vi "ScanPath.vi"(0 "Scan parameters":T2, 1 "Axis parameters":cluster{"X axis":dbl[], "Z axis":dbl[]}={"X axis"=[1.0, 0.0, 0.0], "Z axis"=[0.0, 0.0, 1.0]}, 2 "Position":dbl[](array[numeric]), 3 "error in (no error)":errorcluster) -> (4 "Scanmode":enum16{"X", "Y", "Z", "YZ", "XZ", "XY"}(ring), 5 "ScanPath":T1, 6 "Scan Ready":bool, 7 "Ticks":dbl[][](array[numeric]), 8 "error out":errorcluster)   [LabVIEW 2016]
uses:
  <vilib>/Analysis/Matrix/Datatypes/RealMatrix.ctl
  <vilib>/Analysis/Matrix/NI_Matrix.lvlib
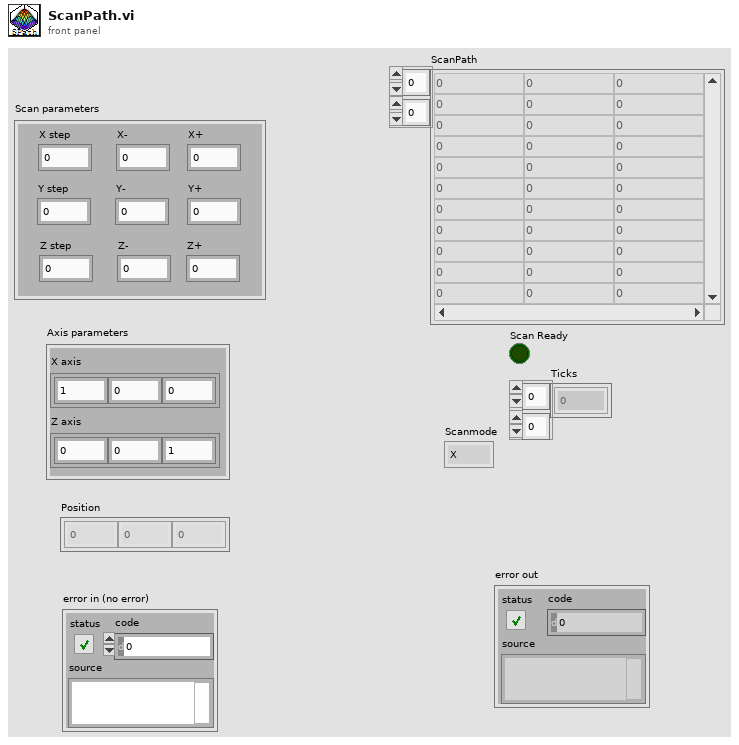
[diagram p1: front panel]
types:
  T1 = typedef "NI_Matrix.lvlib/RealMatrix.ctl" = dbl[][]
  T2 = cluster{"X-":dbl, "X step":dbl, "Y-":dbl, "Y step":dbl, "Z-":dbl, "Z step":dbl, "Z+":dbl, "X+":dbl, "Y+":dbl}
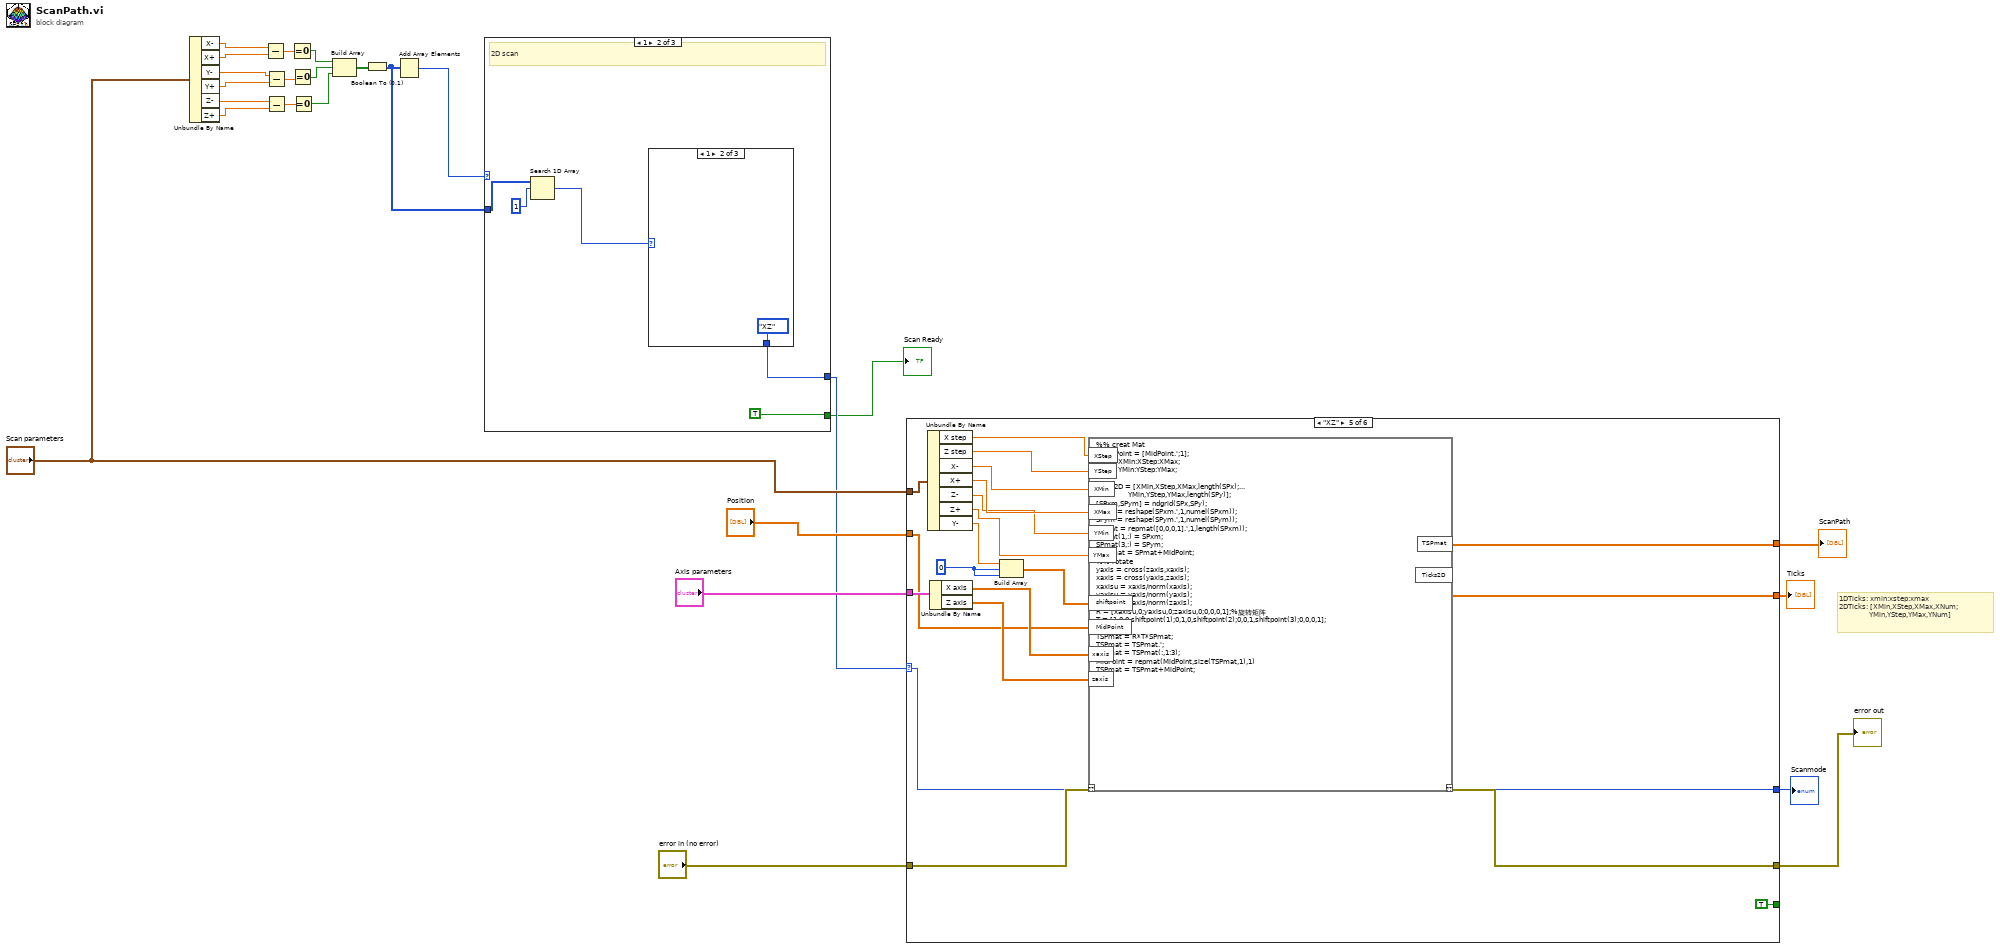
[diagram p0: block diagram]
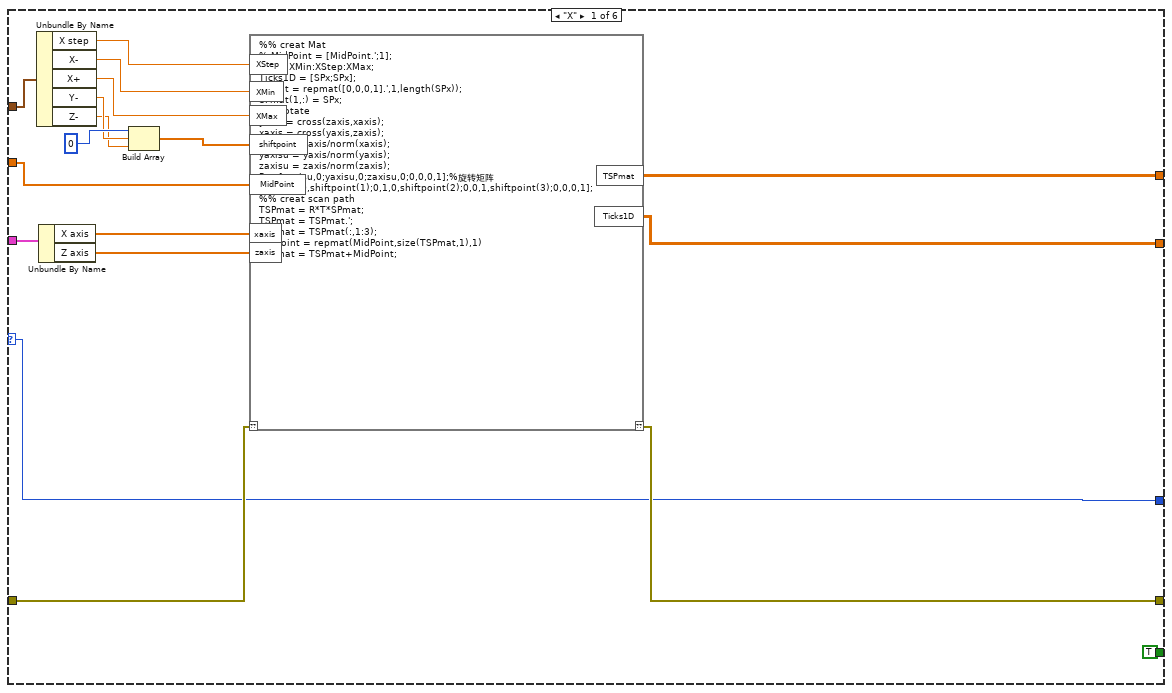
[diagram p2: hidden frame]
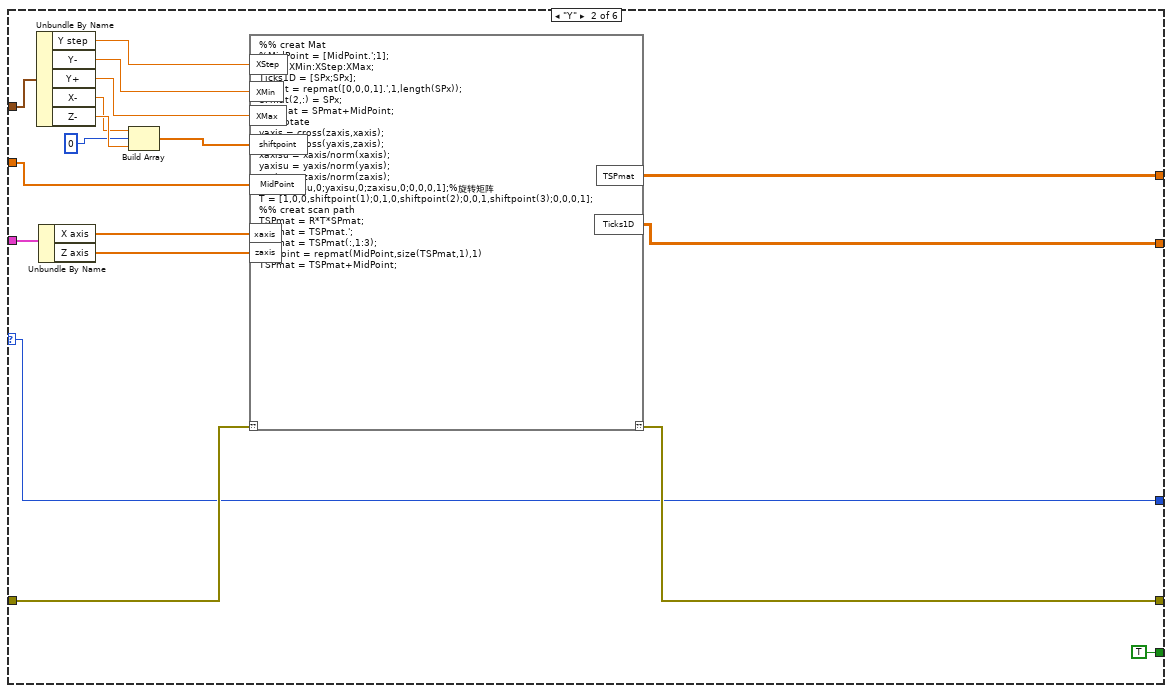
[diagram p3: hidden frame]
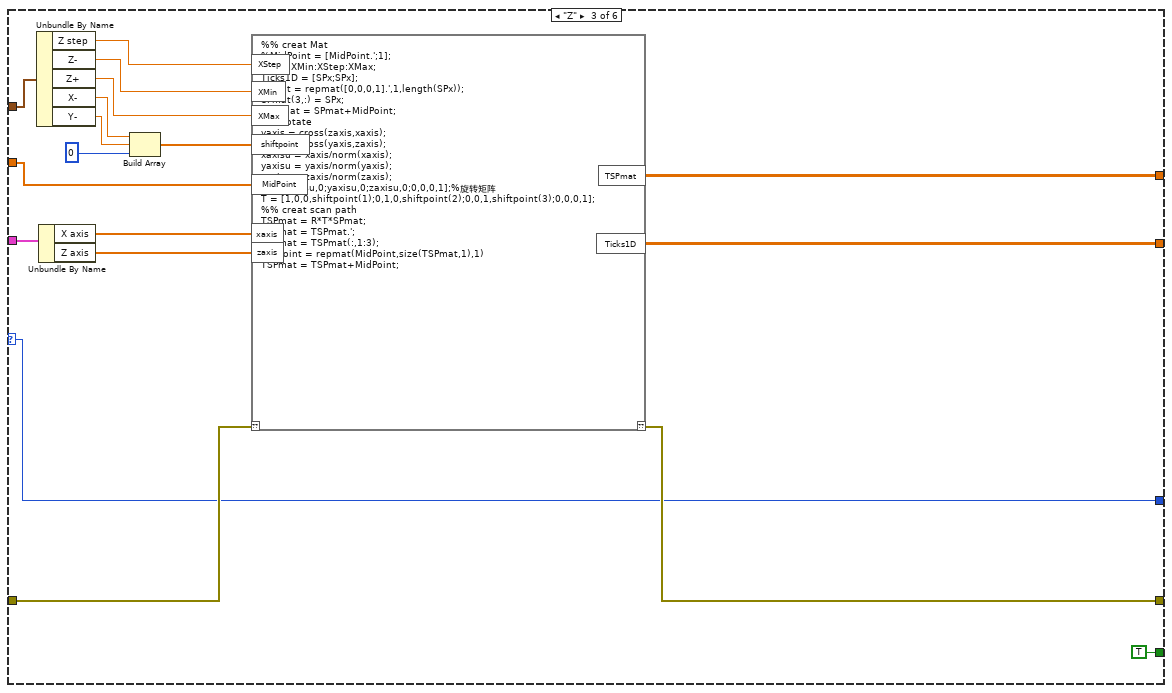
[diagram p4: hidden frame]
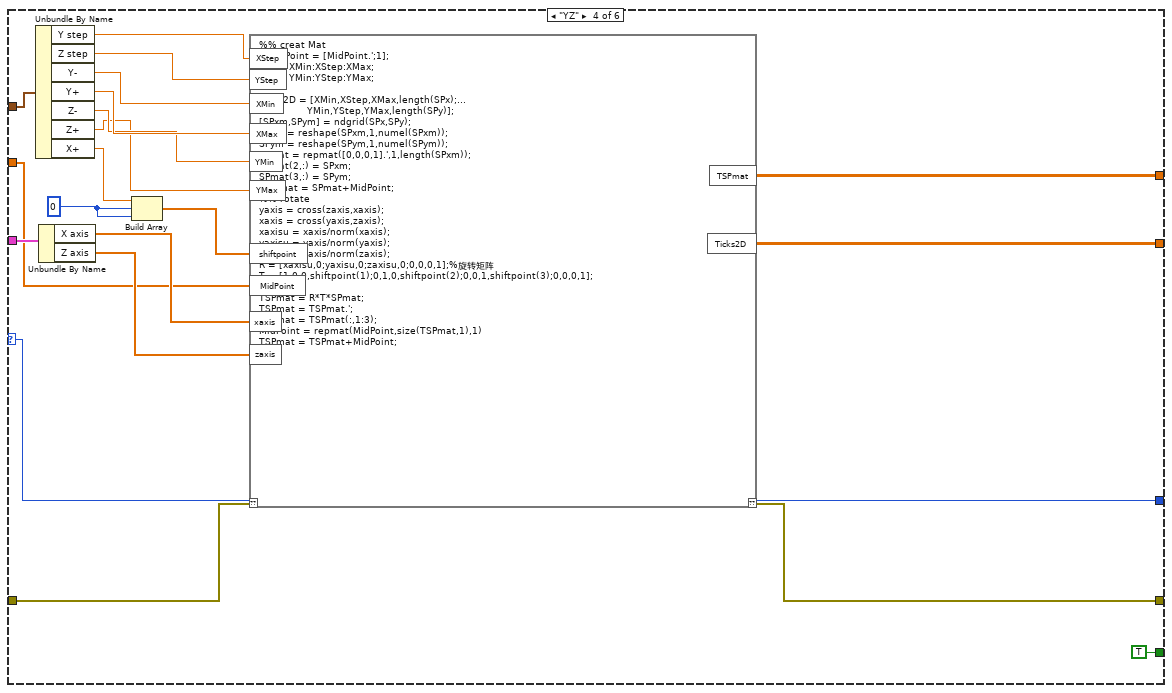
[diagram p5: hidden frame]
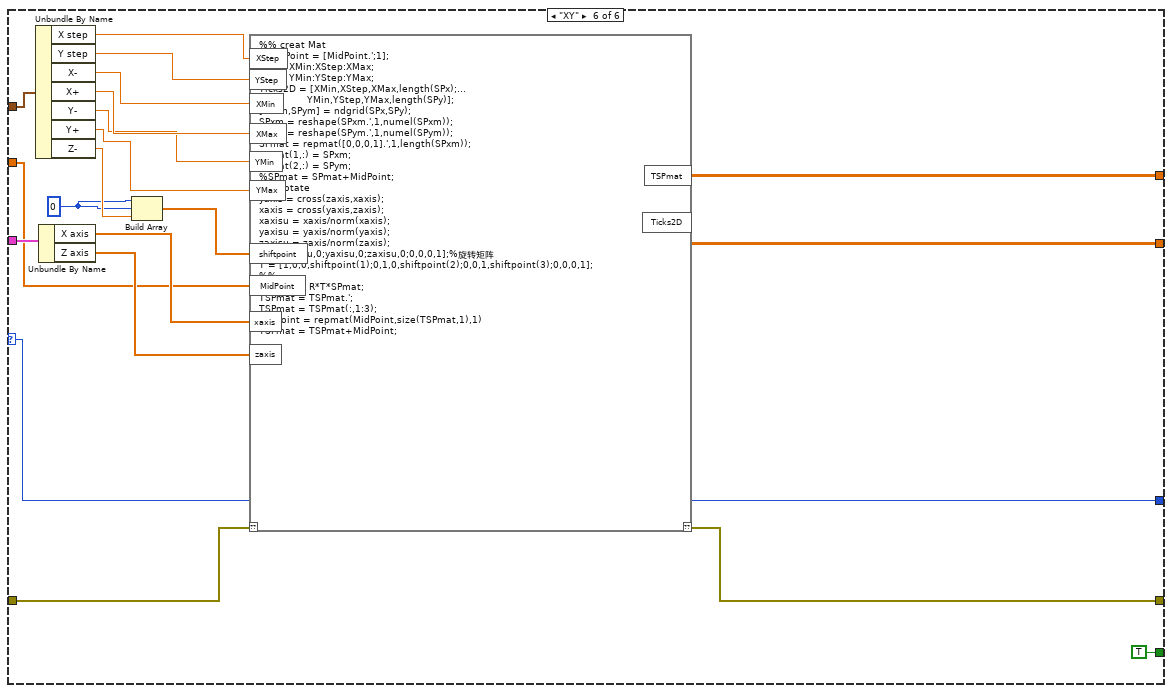
[diagram p6: hidden frame]
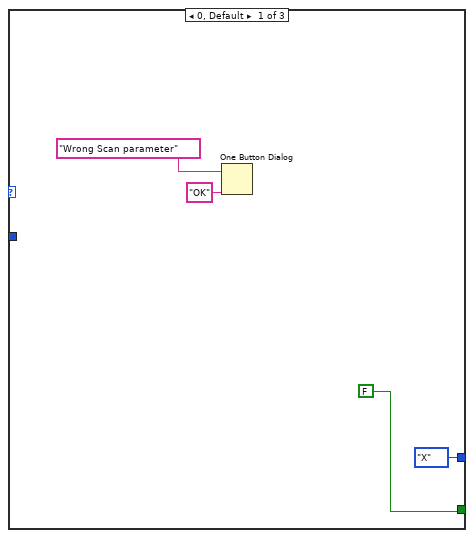
[diagram p7: hidden frame]
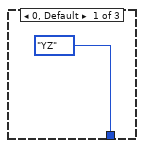
[diagram p8: hidden frame]
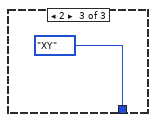
[diagram p9: hidden frame]
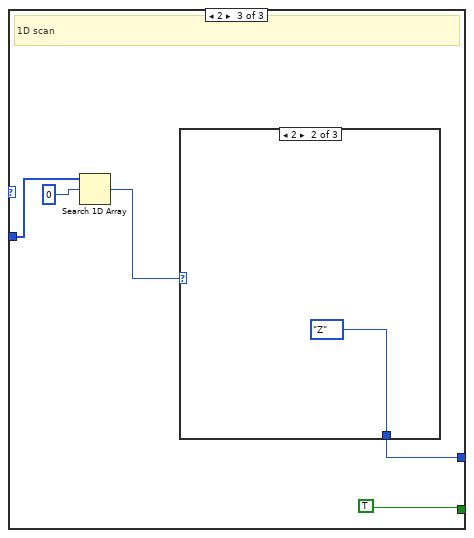
[diagram p10: hidden frame]
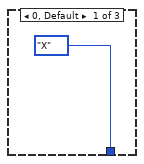
[diagram p11: hidden frame]
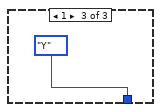
[diagram p12: hidden frame]
diagram:
  # "1DTicks: xmin:xstep:xmax\n2DTicks: [XMin,XStep,XMax,XNum;\n               YMin,YStep,YMax,YNum]"
  n1 = Unbundle By Name("Scan parameters") -> ("X-"=w21:dbl, "X+"=w20:dbl, "Y-"=w19:dbl, "Y+"=w18:dbl, "Z-"=w17:dbl, "Z+"=w16:dbl)
  n2 = Subtract(x=w21, y=w20) -> (x-y=w15:dbl)
  n3 = Subtract(x=w19, y=w18) -> (x-y=w14:dbl)
  n4 = Subtract(x=w17, y=w16) -> (x-y=w13:dbl)
  n5 = Equal To 0?(x=w15) -> (x = 0?=w10:bool)
  n6 = Equal To 0?(x=w14) -> (x = 0?=w12:bool)
  n7 = Equal To 0?(x=w13) -> (x = 0?=w11:bool)
  n8 = Build Array(w10, w12, w11) -> (w9:bool[])
  n9 = Boolean To (0,1)(Boolean=w9) -> (0, 1=w7:i16[])
  n10 = Add Array Elements(numeric array=w7) -> (sum=w8:i16)
  n11 = case shown="1" w8 {
    tunnel: [FALSE TRUE TRUE] -> w3
    tunnel: w7 -> [_ w33 w41]
    tunnel: [enum16{"X", "Y", "Z", "YZ", "XZ", "XY"}."X" w30 w38] -> w5
    frame 0, Default {
      n12 = One Button Dialog(message="Wrong Scan parameter", button name ("OK")="OK") -> ()  [unwired: 1 out]
    }
    frame 1 {
      # "2D scan"
      n13 = Search 1D Array(1D array=w33, element=i16 1) -> (index of element=w31:i32)  [unwired: 1 in]
      n14 = case shown="1" w31 {
        tunnel: [enum16{"X", "Y", "Z", "YZ", "XZ", "XY"}."YZ" enum16{"X", "Y", "Z", "YZ", "XZ", "XY"}."XZ" enum16{"X", "Y", "Z", "YZ", "XZ", "XY"}."XY"] -> w30
        frame 0, Default {
        }
        frame 1 {
        }
        frame 2 {
        }
      }
    }
    frame 2 {
      # "1D scan"
      n15 = Search 1D Array(1D array=w41, element=i16 0) -> (index of element=w39:i32)  [unwired: 1 in]
      n16 = case shown="2" w39 {
        tunnel: [enum16{"X", "Y", "Z", "YZ", "XZ", "XY"}."X" enum16{"X", "Y", "Z", "YZ", "XZ", "XY"}."Z" enum16{"X", "Y", "Z", "YZ", "XZ", "XY"}."Y"] -> w38
        frame 0, Default {
        }
        frame 2 {
        }
        frame 1 {
        }
      }
    }
  }
  "Scan Ready" <- w3
  n17 = case shown="\"XZ\"" w5 {
    selector: w5 -> [w47 w65 w83 w101 w121 w141]
    tunnel: "Scan parameters" -> [w63 w81 w99 w119 w139 w159]
    tunnel: [TRUE TRUE TRUE TRUE TRUE TRUE] -> _
    tunnel: [w47 w65 w83 w101 w121 w141] -> w4
    tunnel: "Position" -> [w51 w71 w90 w111 w131 w151]
    tunnel: "Axis parameters" -> [w59 w77 w95 w116 w136 w156]
    tunnel: "error in (no error)" -> [w53 w73 w92 w113 w133 w153]
    tunnel: [w52 w72 w91 w112 w132 w152] -> w2
    tunnel: [w49 w69 w88 w109 w129 w149] -> w22
    tunnel: [w46 w64 w82 w100 w120 w140] -> w1
    frame "X" {
      n18 = Unbundle By Name(w63) -> ("X step"=w62:dbl, "X-"=w61:dbl, "X+"=w60:dbl, "Y-"=w55:dbl, "Z-"=w54:dbl)
      n19 = Unbundle By Name(w59) -> ("X axis"=w58:dbl[], "Z axis"=w57:dbl[])
      n20 = Build Array(0, w55, w54) -> (w50:dbl[])
      n21 = script code="%% creat Mat\n% MidPoint = [MidPoint.';1];\nSPx = XMin:XStep:XMax;\nTicks1D = [SPx;SPx];\nSPmat = repmat([0,0,0,1].',1,length(SPx));\nSPmat(1,:) = SPx;\n%% rotate \nyaxis = cross(zaxis,xaxis);\nxaxis = cross(yaxis,zaxis);\nxaxisu = xaxis/norm(xaxis);\nyaxisu = yaxis/norm(yaxis);\nzaxisu = zaxis/norm(zaxis);\nR = [xaxisu,0;yaxisu,0;zaxisu,0;0,0,0,1];%旋转矩阵\nT = [1,0,0,shiftpoint(1);0,1,0,shiftpoint(2);0,0,1,shiftpoint(3);0,0,0,1];\n%% creat scan path\nTSPmat = R*T*SPmat;\nTSPmat = TSPmat.';\nTSPmat = TSPmat(:,1:3);\nMidPoint = repmat(MidPoint,size(TSPmat,1),1)\nTSPmat = TSPmat+MidPoint;"("??"=w53, "MidPoint"=w51, "XStep"=w62, "XMin"=w61, "XMax"=w60, "xaxis"=w58, "zaxis"=w57, "shiftpoint"=w50) -> ("??"=w52:errorcluster, "TSPmat"=w49:dbl[][], "Ticks1D"=w46:dbl[][])
    }
    frame "Y" {
      n22 = Unbundle By Name(w81) -> ("Y step"=w80:dbl, "Y-"=w79:dbl, "Y+"=w78:dbl, "X-"=w67:dbl, "Z-"=w74:dbl)
      n23 = Unbundle By Name(w77) -> ("X axis"=w76:dbl[], "Z axis"=w75:dbl[])
      n24 = Build Array(w67, 0, w74) -> (w70:dbl[])
      n25 = script code="%% creat Mat\n%MidPoint = [MidPoint.';1];\nSPx = XMin:XStep:XMax;\nTicks1D = [SPx;SPx];\nSPmat = repmat([0,0,0,1].',1,length(SPx));\nSPmat(2,:) = SPx;\n%SPmat = SPmat+MidPoint;\n%% rotate \nyaxis = cross(zaxis,xaxis);\nxaxis = cross(yaxis,zaxis);\nxaxisu = xaxis/norm(xaxis);\nyaxisu = yaxis/norm(yaxis);\nzaxisu = zaxis/norm(zaxis);\nR = [xaxisu,0;yaxisu,0;zaxisu,0;0,0,0,1];%旋转矩阵\nT = [1,0,0,shiftpoint(1);0,1,0,shiftpoint(2);0,0,1,shiftpoint(3);0,0,0,1];\n%% creat scan path\nTSPmat = R*T*SPmat;\nTSPmat = TSPmat.';\nTSPmat = TSPmat(:,1:3);\nMidPoint = repmat(MidPoint,size(TSPmat,1),1)\nTSPmat = TSPmat+MidPoint;"("??"=w73, "MidPoint"=w71, "XStep"=w80, "XMin"=w79, "XMax"=w78, "xaxis"=w76, "zaxis"=w75, "shiftpoint"=w70) -> ("??"=w72:errorcluster, "TSPmat"=w69:dbl[][], "Ticks1D"=w64:dbl[][])
    }
    frame "Z" {
      n26 = Unbundle By Name(w99) -> ("Z step"=w98:dbl, "Z-"=w97:dbl, "Z+"=w96:dbl, "X-"=w87:dbl, "Y-"=w84:dbl)
      n27 = Unbundle By Name(w95) -> ("X axis"=w94:dbl[], "Z axis"=w93:dbl[])
      n28 = Build Array(w87, w84, 0) -> (w89:dbl[])
      n29 = script code="%% creat Mat\n%MidPoint = [MidPoint.';1];\nSPx = XMin:XStep:XMax;\nTicks1D = [SPx;SPx];\nSPmat = repmat([0,0,0,1].',1,length(SPx));\nSPmat(3,:) = SPx;\n%SPmat = SPmat+MidPoint;\n%% rotate \nyaxis = cross(zaxis,xaxis);\nxaxis = cross(yaxis,zaxis);\nxaxisu = xaxis/norm(xaxis);\nyaxisu = yaxis/norm(yaxis);\nzaxisu = zaxis/norm(zaxis);\nR = [xaxisu,0;yaxisu,0;zaxisu,0;0,0,0,1];%旋转矩阵\nT = [1,0,0,shiftpoint(1);0,1,0,shiftpoint(2);0,0,1,shiftpoint(3);0,0,0,1];\n%% creat scan path\nTSPmat = R*T*SPmat;\nTSPmat = TSPmat.';\nTSPmat = TSPmat(:,1:3);\nMidPoint = repmat(MidPoint,size(TSPmat,1),1)\nTSPmat = TSPmat+MidPoint;"("??"=w92, "MidPoint"=w90, "XStep"=w98, "XMin"=w97, "XMax"=w96, "xaxis"=w94, "zaxis"=w93, "shiftpoint"=w89) -> ("??"=w91:errorcluster, "TSPmat"=w88:dbl[][], "Ticks1D"=w82:dbl[][])
    }
    frame "YZ" {
      w106 = 0
      n30 = Unbundle By Name(w119) -> ("Y step"=w102:dbl, "Z step"=w103:dbl, "Y-"=w118:dbl, "Y+"=w117:dbl, "Z-"=w105:dbl, "Z+"=w104:dbl, "X+"=w107:dbl)
      n31 = Unbundle By Name(w116) -> ("X axis"=w115:dbl[], "Z axis"=w114:dbl[])
      n32 = Build Array(w107, w106, w106) -> (w110:dbl[])
      n33 = script code="%% creat Mat\n%MidPoint = [MidPoint.';1];\nSPx = XMin:XStep:XMax;\nSPy = YMin:YStep:YMax;\n\nTicks2D = [XMin,XStep,XMax,length(SPx);...\n                YMin,YStep,YMax,length(SPy)];\n[SPxm,SPym] = ndgrid(SPx,SPy);\nSPxm = reshape(SPxm,1,numel(SPxm));\nSPym = reshape(SPym,1,numel(SPym));\nSPmat = repmat([0,0,0,1].',1,length(SPxm));\nSPmat(2,:) = SPxm;\nSPmat(3,:) = SPym;\n%SPmat = SPmat+MidPoint;\n%% rotate \nyaxis = cross(zaxis,xaxis);\nxaxis = cross(yaxis,zaxis);\nxaxisu = xaxis/norm(xaxis);\nyaxisu = yaxis/norm(yaxis);\nzaxisu = zaxis/norm(zaxis);\nR = [xaxisu,0;yaxisu,0;zaxisu,0;0,0,0,1];%旋转矩阵\nT = [1,0,0,shiftpoint(1);0,1,0,shiftpoint(2);0,0,1,shiftpoint(3);0,0,0,1];\n%%\nTSPmat = R*T*SPmat;\nTSPmat = TSPmat.';\nTSPmat = TSPmat(:,1:3);\nMidPoint = repmat(MidPoint,size(TSPmat,1),1)\nTSPmat = TSPmat+MidPoint;"("??"=w113, "MidPoint"=w111, "XStep"=w102, "XMin"=w118, "XMax"=w117, "xaxis"=w115, "zaxis"=w114, "shiftpoint"=w110, "YMin"=w105, "YMax"=w104, "YStep"=w103) -> ("??"=w112:errorcluster, "TSPmat"=w109:dbl[][], "Ticks2D"=w100:dbl[][])
    }
    frame "XZ" {
      w126 = 0
      n34 = Unbundle By Name(w139) -> ("X step"=w122:dbl, "Z step"=w123:dbl, "X-"=w138:dbl, "X+"=w137:dbl, "Z-"=w125:dbl, "Z+"=w124:dbl, "Y-"=w127:dbl)
      n35 = Unbundle By Name(w136) -> ("X axis"=w135:dbl[], "Z axis"=w134:dbl[])
      n36 = Build Array(w127, w126, w126) -> (w130:dbl[])
      n37 = script code="%% creat Mat\n%MidPoint = [MidPoint.';1];\nSPx = XMin:XStep:XMax;\nSPy = YMin:YStep:YMax;\n\nTicks2D = [XMin,XStep,XMax,length(SPx);...\n                YMin,YStep,YMax,length(SPy)];\n[SPxm,SPym] = ndgrid(SPx,SPy);\nSPxm = reshape(SPxm.',1,numel(SPxm));\nSPym = reshape(SPym.',1,numel(SPym));\nSPmat = repmat([0,0,0,1].',1,length(SPxm));\nSPmat(1,:) = SPxm;\nSPmat(3,:) = SPym;\n%SPmat = SPmat+MidPoint;\n%% rotate \nyaxis = cross(zaxis,xaxis);\nxaxis = cross(yaxis,zaxis);\nxaxisu = xaxis/norm(xaxis);\nyaxisu = yaxis/norm(yaxis);\nzaxisu = zaxis/norm(zaxis);\nR = [xaxisu,0;yaxisu,0;zaxisu,0;0,0,0,1];%旋转矩阵\nT = [1,0,0,shiftpoint(1);0,1,0,shiftpoint(2);0,0,1,shiftpoint(3);0,0,0,1];\n%%\nTSPmat = R*T*SPmat;\nTSPmat = TSPmat.';\nTSPmat = TSPmat(:,1:3);\nMidPoint = repmat(MidPoint,size(TSPmat,1),1)\nTSPmat = TSPmat+MidPoint;"("??"=w133, "MidPoint"=w131, "XStep"=w122, "XMin"=w138, "XMax"=w137, "xaxis"=w135, "zaxis"=w134, "shiftpoint"=w130, "YMin"=w125, "YMax"=w124, "YStep"=w123) -> ("??"=w132:errorcluster, "TSPmat"=w129:dbl[][], "Ticks2D"=w120:dbl[][])
    }
    frame "XY" {
      w142 = 0
      n38 = Unbundle By Name(w159) -> ("X step"=w144:dbl, "Y step"=w145:dbl, "X-"=w158:dbl, "X+"=w157:dbl, "Y-"=w147:dbl, "Y+"=w146:dbl, "Z-"=w143:dbl)
      n39 = Unbundle By Name(w156) -> ("X axis"=w155:dbl[], "Z axis"=w154:dbl[])
      n40 = Build Array(w142, w142, w143) -> (w150:dbl[])
      n41 = script code="%% creat Mat\n%MidPoint = [MidPoint.';1];\nSPx = XMin:XStep:XMax;\nSPy = YMin:YStep:YMax;\nTicks2D = [XMin,XStep,XMax,length(SPx);...\n                YMin,YStep,YMax,length(SPy)];\n[SPxm,SPym] = ndgrid(SPx,SPy);\nSPxm = reshape(SPxm.',1,numel(SPxm));\nSPym = reshape(SPym.',1,numel(SPym));\nSPmat = repmat([0,0,0,1].',1,length(SPxm));\nSPmat(1,:) = SPxm;\nSPmat(2,:) = SPym;\n%SPmat = SPmat+MidPoint;\n%% rotate \nyaxis = cross(zaxis,xaxis);\nxaxis = cross(yaxis,zaxis);\nxaxisu = xaxis/norm(xaxis);\nyaxisu = yaxis/norm(yaxis);\nzaxisu = zaxis/norm(zaxis);\nR = [xaxisu,0;yaxisu,0;zaxisu,0;0,0,0,1];%旋转矩阵\nT = [1,0,0,shiftpoint(1);0,1,0,shiftpoint(2);0,0,1,shiftpoint(3);0,0,0,1];\n%%\nTSPmat = R*T*SPmat;\nTSPmat = TSPmat.';\nTSPmat = TSPmat(:,1:3);\nMidPoint = repmat(MidPoint,size(TSPmat,1),1)\nTSPmat = TSPmat+MidPoint;"("??"=w153, "MidPoint"=w151, "XStep"=w144, "XMin"=w158, "XMax"=w157, "xaxis"=w155, "zaxis"=w154, "shiftpoint"=w150, "YMin"=w147, "YMax"=w146, "YStep"=w145) -> ("??"=w152:errorcluster, "TSPmat"=w149:dbl[][], "Ticks2D"=w140:dbl[][])
    }
  }
  "error out" <- w2
  "ScanPath" <- w22
  "Scanmode" <- w4
  "Ticks" <- w1
